vi "Create Rect Array.vi"() -> (3 "矩形数组":refnum<class "矩形.lvclass">[](array[class]))   [LabVIEW 2013, in "矩形.lvclass"]
panel:
  out "error out":errorcluster caption="错误输出"
  in  "error in (no error)":errorcluster caption="错误输入（无错误）"
  in  "宽度":dbl[](array[numeric])
  in  "长度":dbl[](array[numeric])
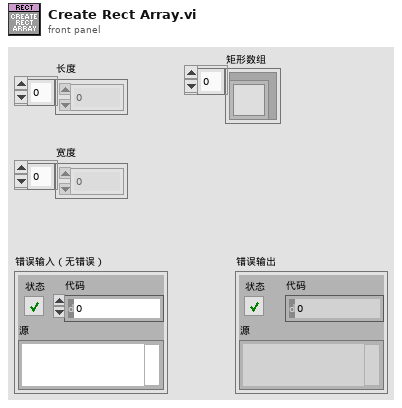
[diagram p1: front panel]
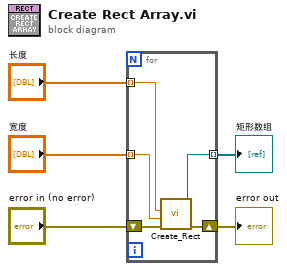
[diagram p0: block diagram]
diagram:
  n1 = for {
    tunnel: "长度" -> [w8] mode=indexing
    tunnel: "宽度" -> [w7] mode=indexing
    shift-right: [w9] -> w2
    shift-left: "error in (no error)" -> [w10]
    tunnel: [w6] -> w1 mode=indexing
    n2 = call "Create_Rect.vi"("error in (no error)"=w10, "宽度"=w7, "长度"=w8) -> ("error out"=w9:errorcluster, "矩形类 输出"=w6:refnum<class "矩形.lvclass">)  [unwired: 7 in]
  }
  "error out" <- w2
  "矩形数组" <- w1
